vi "drawCells.vi"(8 "error in":errorcluster, 9 "diameter (px)":i32=100, 10 "current cell locations (px)":dbl[][](array[numeric]), 11 "Image in":T1) -> (0 "error out":errorcluster, 3 "Image out":T1)   [LabVIEW 2015]
uses:
  <vilib>/vision/Image Controls.llb/IMAQ Image.ctl
panel:
  # "DRAW CELLS"
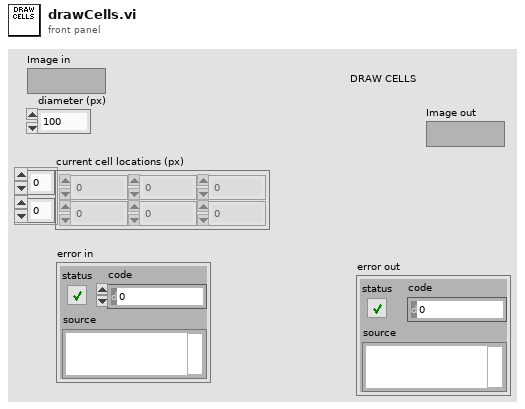
[diagram p1: front panel]
types:
  T1 = typedef "IMAQ Image.ctl" = refnum<image>
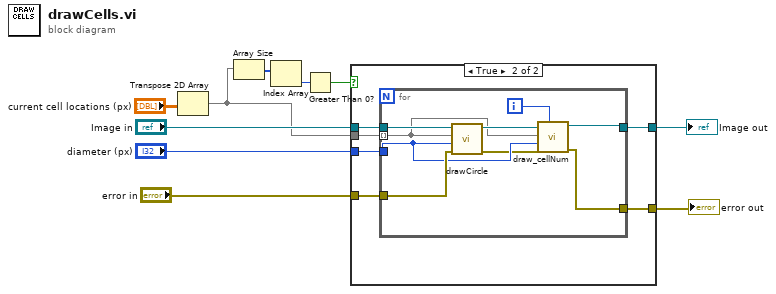
[diagram p0: block diagram]
diagram:
  n1 = Transpose 2D Array(2D array="current cell locations (px)") -> (transposed array=w4:dbl[][])
  n2 = Array Size(array=w4) -> (size(s)=w3:i32[])
  n3 = Index Array(array=w3) -> (element=w2:i32)  [unwired: 1 in]
  n4 = Greater Than 0?(x=w2) -> (x > 0?=w1:bool)
  n5 = case shown="True" w1 {
    tunnel: "Image in" -> [w12 w18]
    tunnel: "diameter (px)" -> [_ w17]
    tunnel: [w12 w16] -> w8
    tunnel: "error in" -> [w11 w15]
    tunnel: [w11 w14] -> w6
    tunnel: w4 -> [_ w13]
    frame False {
    }
    frame True {
      n6 = for {
        tunnel: w18 -> [w27]
        tunnel: w13 -> [w24] mode=indexing
        tunnel: w17 -> [w23]
        tunnel: [w19] -> w16
        tunnel: w15 -> [w26]
        tunnel: [w21] -> w14
        i -> [w20]
        n7 = call "drawCircle.vi"("error in"=w26, "diameter"=w23, "center (x,y)"=w24, "Image in"=w27) -> ("error out"=w22:errorcluster, "Image out"=w25:T1)  [unwired: 6 in]
        n8 = call "draw_cellNum.vi"("cell index"=w20, "error in"=w22, "diameter (px)"=w23, "center (x,y)"=w24, "Image in"=w25) -> ("error out"=w21:errorcluster, "Image out"=w19:T1)  [unwired: 5 in]
      }
    }
  }
  "Image out" <- w8
  "error out" <- w6
